vi "value to value(limit).vi"(8 "high limit":dbl, 9 "low limit":dbl, 11 "数值 in":dbl) -> (3 "数值 out":dbl)   [LabVIEW 2019, in "SubVI.lvlib"]
uses:
  SubVI.lvlib
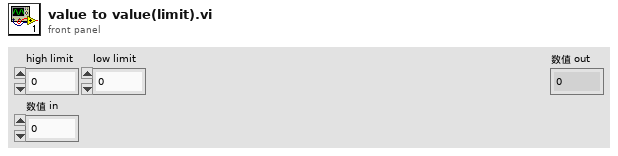
[diagram p1: front panel]
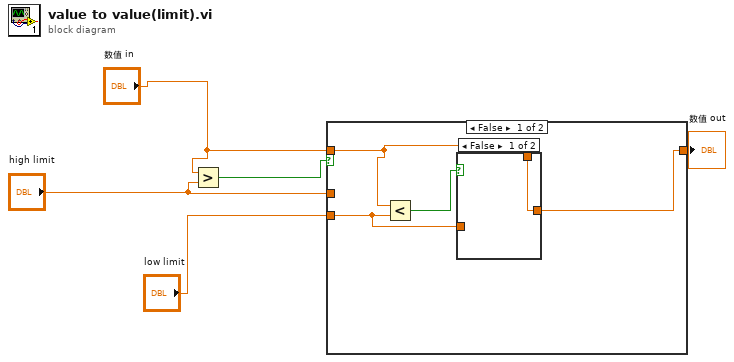
[diagram p0: block diagram]
diagram:
  n1 = Greater?(x="数值 in", y="high limit") -> (0:w5:bool)
  n2 = case shown="False" w5 {
    tunnel: "数值 in" -> [w6 _]
    tunnel: [w7 w12] -> w4
    tunnel: "high limit" -> [_ w12]
    tunnel: "low limit" -> [w8 _]
    frame False {
      n3 = Less?(x=w6, y=w8) -> (x < y?=w9:bool)
      n4 = case shown="False" w9 {
        tunnel: w8 -> [_ w11]
        tunnel: [w10 w11] -> w7
        tunnel: w6 -> [w10 _]
        frame False {
        }
        frame True {
        }
      }
    }
    frame True {
    }
  }
  "数值 out" <- w4
